vi "calc_phase.vi"(11 "phase [rad]":dbl) -> (3 "phase":dbl)   [LabVIEW 2025]
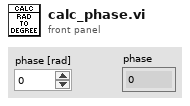
[diagram p1: front panel]
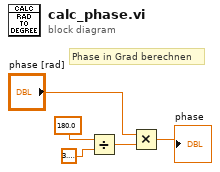
[diagram p0: block diagram]
diagram:
  # "Phase in Grad berechnen"
  n1 = Divide(x=180.0, y=3.141592653589793) -> (x/y=w4:dbl)
  n2 = Multiply(x="phase [rad]", y=w4) -> (x*y=→"phase":dbl)
